vi "RequestAndTrace.vi"(0 "JSONRef in":T1, 1 "TraceRef":refnum<vi>, 5 "method":string, 7 "params":refnum<class "JSON Null.lvclass">, 11 "error in (no error)":errorcluster) -> (4 "JSONRef out":T1, 6 "reponse":string, 15 "error out":errorcluster)   [LabVIEW 2017]
uses:
  jsonRPCwebservice/client/reference.ctl
  <vilib>/httpClient/ClientHandle.ctl
  <vilib>/NI/JSON Support for LabVIEW/JSON Data Classes/JSON Datatype/JSON Null.lvclass
  jsonRPCwebservice/client/Request_int_str.vi
  jsonRPCwebservice/client/JSON_RPC_client.lvlib
  <vilib>/httpClient/LabVIEWHTTPClient.lvlib
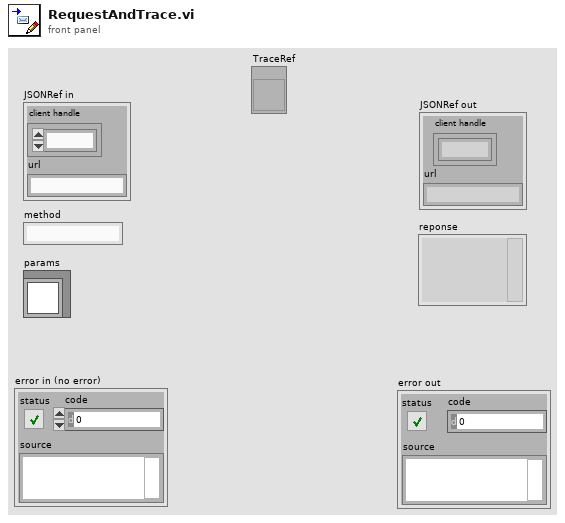
[diagram p1: front panel]
types:
  T1 = typedef "JSON_RPC_client.lvlib/reference.ctl" = cluster{"client handle":T2, "url":string}
  T2 = typedef "LabVIEWHTTPClient.lvlib/ClientHandle.ctl" = refnum<k1>
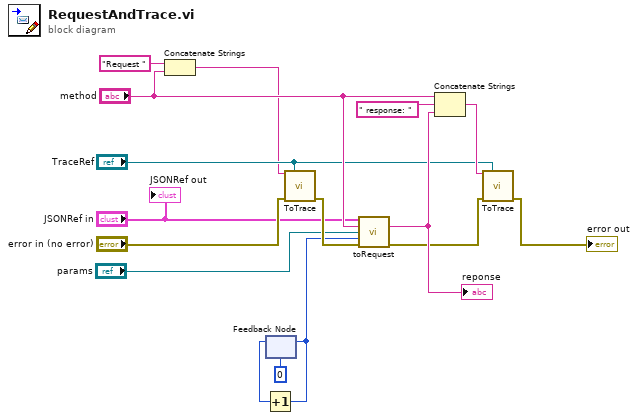
[diagram p0: block diagram]
diagram:
  n1 = Concatenate Strings("Request ", "method") -> (w9:string)
  n2 = feedback #1(0 ("id")) -> (w3:i32)
  n3 = Increment(x=w3) -> (x+1=w2:i32)
  n4 = feedback-in #1(w2) -> ()
  n5 = call "ToTrace.vi"("ToTrace"=w9, "TraceRef"="TraceRef", "error in (no error)"="error in (no error)") -> ("error out"=w7:errorcluster)  [unwired: 12 in]
  n6 = call-poly "toRequest.vi"("reference in"="JSONRef in", "method"="method", "params"="params", "id"=w2, "error in (no error)"=w7) -> ("response"=w15:string, "error out"=w11:errorcluster)  [unwired: 8 in, 1 out]
  "reponse" <- w15
  n7 = Concatenate Strings("method", " response: " ("string"), w15) -> (w16:string)
  n8 = call "ToTrace.vi"("ToTrace"=w16, "TraceRef"="TraceRef", "error in (no error)"=w11) -> ("error out"=→"error out":errorcluster)  [unwired: 12 in]
  "JSONRef out" <- "JSONRef in"
